vi "Get Scaling Parameters (Polynomial).vi"(0 "session in":refnum<k21>, 5 "physical channel":refnum<k21>="$DefaultPhysChans", 11 "error in (no error)":errorcluster) -> (4 "session out":refnum<k21>, 6 "physical channel out":refnum<k21>, 8 "forward coefficients":dbl[](array[numeric]), 10 "reverse coefficients":dbl[](array[numeric]), 15 "error out":errorcluster)   [LabVIEW 2020, in "SLSC.lvlib"]
doc: "Gets scaling parameters from a polynomial scale that uses an nth order polynomial equation. A polynomial scale contains both a polynomial to convert pre-scaled values to scaled values and a polynomial to convert scaled values to pre-scaled values."
uses:
  <vilib>/SLSC/SLSC.lvlib
  nislsclvapi.dll
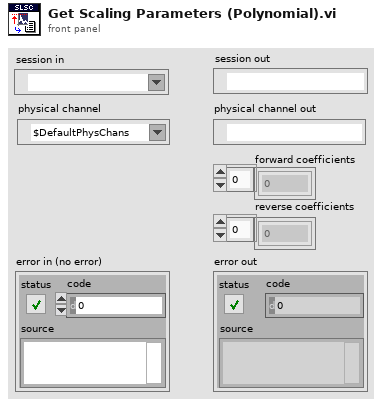
[diagram p1: front panel]
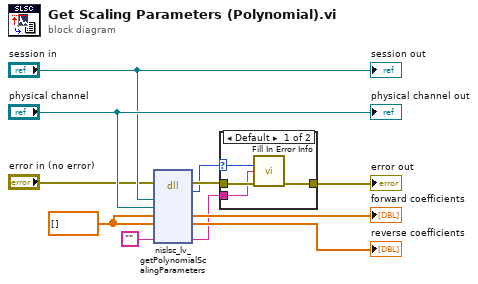
[diagram p0: block diagram]
diagram:
  w10 = dbl[] [] ("forwardCoeffs")
  n1 = dll-call lib="nislsclvapi.*" fn="nislsc_lv_getPolynomialScalingParameters"(error in="error in (no error)", "session"="session in", "physical channel"="physical channel", "forwardCoeffs"=w10, "reverseCoeffs"=w10, "extendedErrorInfo"="") -> (error out=w3:errorcluster, "return type"=w1:i32, "forwardCoeffs"=→"forward coefficients":dbl[], "reverseCoeffs"=→"reverse coefficients":dbl[], "extendedErrorInfo"=w2:string)  [unwired: 6 in, 1 out]
  n2 = case shown="Default" w1 {
    selector: w1 -> [w12 _]
    tunnel: w2 -> [w13 _]
    tunnel: w3 -> [w15 w16]
    tunnel: [w14 w16] -> w4
    frame Default {
      n3 = call <vilib>:"Fill In Error Info.vi"("status code"=w12, "extended error info"=w13, "error in"=w15) -> ("error out"=w14:errorcluster)  [unwired: 12 in]
    }
    frame 0 {
    }
  }
  "error out" <- w4
  "session out" <- "session in"
  "physical channel out" <- "physical channel"
